vi "assign object ID.vi"(3 "object calculations (previous)":T2[](array[typedef]), 4 "robot location":cluster{"x":i16, "y":i16}, 5 "visible objects":T3[](array[typedef])) -> (0 "faulty trailer detection":bool, 2 "IDed objects":T1(array[cluster]))   [LabVIEW 2009]
uses:
  visible object.ctl
  object velocity and calculations.ctl
panel:
  out "checksum 2":i32
  out "checksum 1":i16
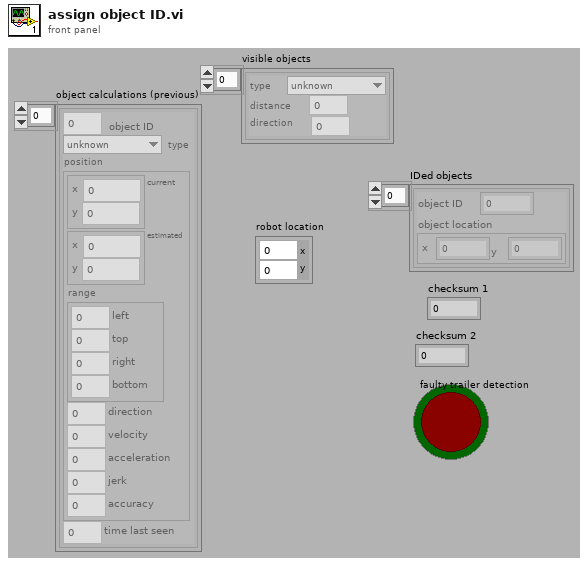
[diagram p1: front panel]
types:
  T1 = cluster{"object ID":i32, "object location":cluster{"x":dbl, "y":dbl}}[]
  T2 = typedef "object velocity and calculations.ctl" = cluster{"object ID":i32, "type":enum8{"unknown", "moonrock", "empty cell", "supercell", "target trailer"}, "position":cluster{"current":cluster{"x":dbl, "y":dbl}, "estimated":cluster{"x":dbl, "y":dbl}, "range":cluster{"left":dbl, "top":dbl, "right":dbl, "bottom":dbl}, "direction":dbl, "velocity":dbl, "acceleration":dbl, "jerk":dbl, "accuracy":dbl}, "time last seen":i32}
  T3 = typedef "visible object.ctl" = cluster{"type":enum8{"unknown", "moonrock", "empty cell", "supercell", "target trailer"}, "distance":dbl, "direction":dbl}
  T4 = enum8{"unknown", "moonrock", "empty cell", "supercell", "target trailer"}
  T5 = cluster{"current":cluster{"x":dbl, "y":dbl}, "estimated":cluster{"x":dbl, "y":dbl}, "range":cluster{"left":dbl, "top":dbl, "right":dbl, "bottom":dbl}, "direction":dbl, "velocity":dbl, "acceleration":dbl, "jerk":dbl, "accuracy":dbl}
  T6 = cluster{"left":dbl, "top":dbl, "right":dbl, "bottom":dbl}
  T7 = cluster{"In Range?":bool, "distance":dbl, i32, cluster{dbl, dbl}}
  T8 = cluster{"In Range?":bool, "distance":dbl, i32, cluster{dbl, dbl}}[]
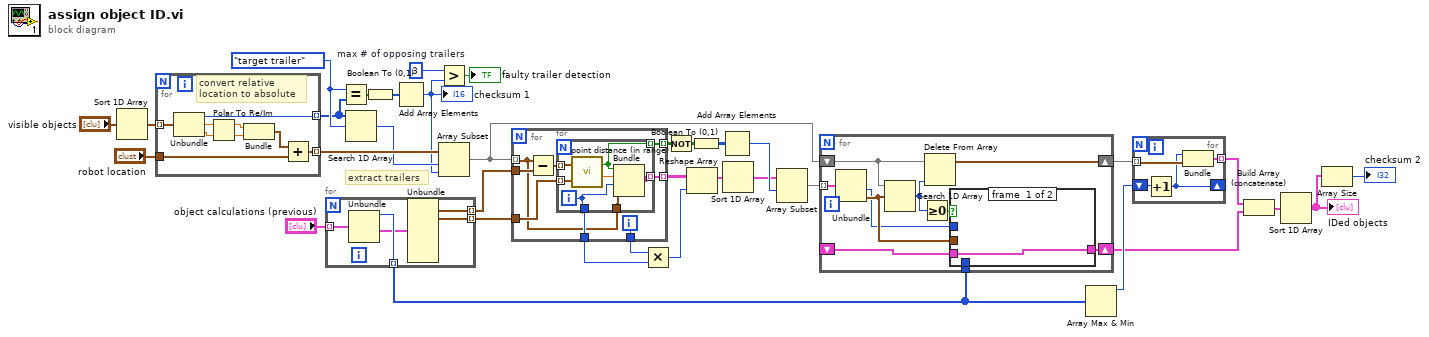
[diagram p0: block diagram]
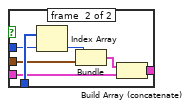
[diagram p2: hidden frame]
diagram:
  w26 = i16 3  # max # of opposing trailers
  w31 = T4."target trailer" ("type")
  # "extract trailers"
  n1 = Sort 1D Array(array="visible objects") -> (sorted array=w33:T3[])
  n2 = for {
    tunnel: w33 -> [w44] mode=indexing
    tunnel: "robot location" -> [w38]
    tunnel: [w37] -> w32 mode=indexing
    tunnel: [w36] -> w30 mode=indexing
    # "convert relative\nlocation to absolute"
    n3 = Unbundle(w44) -> ("type"=w36:T4, "distance"=w43:dbl, "direction"=w42:dbl)
    n4 = Polar To Re/Im(2:w42, 3:w43) -> (0:w41:dbl, 1:w40:dbl)
    n5 = Bundle(w40, w41) -> (w39:cluster{dbl, dbl})  [unwired: 1 in]
    n6 = Add(x=w39, y=w38) -> (x+y=w37:cluster{dbl, dbl})
  }
  n7 = for {
    tunnel: "object calculations (previous)" -> [w49] mode=indexing
    tunnel: [w48] -> w10 mode=indexing
    tunnel: [w46] -> w24 mode=indexing
    tunnel: [w45] -> w23 mode=indexing
    n8 = Unbundle(w49) -> ("object ID"=w48:i32, "position"=w47:T5)  [unwired: 2 out]
    n9 = Unbundle(w47) -> ("estimated"=w46:cluster{"x":dbl, "y":dbl}, "range"=w45:T6)  [unwired: 6 out]
  }
  n10 = Equal?(x=w31, y=w30) -> (x = y?=w29:bool[])
  n11 = Search 1D Array(1D array=w30, element=w31) -> (index of element=w27:i32)  [unwired: 1 in]
  n12 = Boolean To (0,1)(Boolean=w29) -> (0, 1=w28:i16[])
  n13 = Add Array Elements(numeric array=w28) -> (sum=w2:i16)
  "checksum 1" <- w2
  n14 = Greater?(x=w26, y=w2) -> (0:→"faulty trailer detection":bool)
  n15 = Array Subset(array=w32, index=w27, length=w2) -> (w11:cluster{dbl, dbl}[])
  n16 = for {
    tunnel: w11 -> [w50] mode=indexing
    tunnel: w24 -> [w57]
    tunnel: w23 -> [w55]
    tunnel: [w54] -> w20 mode=indexing
    tunnel: [w53] -> w21
    tunnel: [w51] -> w22
    tunnel: [w52] -> w16 mode=indexing
    i -> [w51]
    n17 = Subtract(x=w50, y=w57) -> (x-y=w56:cluster{dbl, dbl}[])
    n18 = for {
      tunnel: w56 -> [w63] mode=indexing
      tunnel: w55 -> [w64] mode=indexing
      tunnel: [w61] -> w54 mode=indexing
      tunnel: [w60] -> w52 mode=indexing
      tunnel: [w59] -> w53
      tunnel: w50 -> [w58]
      i -> [w59]
      n19 = call "point distance (in range).vi"("range"=w64, "cartesian location"=w63) -> ("distance"=w62:dbl, "In Range?"=w60:bool)
      n20 = Bundle("In Range?"=w60, "distance"=w62, w59, w58) -> (w61:T7)  [unwired: 1 in]
    }
  }
  n21 = Multiply(x=w22, y=w21) -> (x*y=w19:i32)
  n22 = Not(x=w16) -> (.not. x?=w18:bool[][])
  n23 = Reshape Array(w20, w19) -> (w15:T8)
  n24 = Boolean To (0,1)(Boolean=w18) -> (0, 1=w17:i16[][])
  n25 = Add Array Elements(numeric array=w17) -> (sum=w14:i16)
  n26 = Sort 1D Array(array=w15) -> (sorted array=w13:T8)
  n27 = Array Subset(array=w13, index=w14) -> (w12:T8)  [unwired: 1 in]
  n28 = for {
    tunnel: w12 -> [w74] mode=indexing
    shift-right: [w72] -> w8
    shift-left: w11 -> [w73]
    tunnel: w10 -> [w68]
    shift-right: [w66] -> w6
    shift-left: _ -> [w65]
    n29 = Unbundle(w74) -> (w67:i32, w69:cluster{dbl, dbl})  [unwired: 2 out]
    n30 = Search 1D Array(1D array=w73, element=w69) -> (index of element=w71:i32)  [unwired: 1 in]
    n31 = Greater Or Equal To 0?(x=w71) -> (x >= 0?=w70:bool)
    n32 = Delete From Array(array=w73, index=w71) -> (array with subset deleted=w72:cluster{dbl, dbl}[])  [unwired: 1 in, 1 out]
    n33 = case shown="True" w70 {
      tunnel: w69 -> [_ w79]
      tunnel: w68 -> [_ w82]
      tunnel: w67 -> [_ w81]
      tunnel: [w75 w77] -> w66
      tunnel: w65 -> [w75 w76]
      frame #0 {
      }
      frame #1 {
        n34 = Index Array(array=w82, index=w81) -> (element=w80:i32)
        n35 = Bundle("object ID"=w80, w79) -> (w78:cluster{"object ID":i32, cluster{dbl, dbl}})  [unwired: 1 in]
        n36 = Build Array (concatenate)(w78, w76) -> (w77:cluster{"object ID":i32, cluster{dbl, dbl}}[])
      }
    }
  }
  n37 = Array Max & Min(array=w10) -> (max value=w9:i32)  [unwired: 3 out]
  n38 = for {
    shift-right: [w84] -> _
    shift-left: w9 -> [w86]
    tunnel: w8 -> [w85] mode=indexing
    tunnel: [w83] -> w7 mode=indexing
    n39 = Increment(x=w86) -> (x+1=w84:i32)
    n40 = Bundle(w84, w85) -> (w83:cluster{i32, cluster{dbl, dbl}})  [unwired: 1 in]
  }
  n41 = Build Array (concatenate)(w7, w6) -> (w5:cluster{"object ID":i32, cluster{dbl, dbl}}[])
  n42 = Sort 1D Array(array=w5) -> (sorted array=w4:cluster{"object ID":i32, cluster{dbl, dbl}}[])
  "IDed objects" <- w4
  n43 = Array Size(array=w4) -> (size(s)=→"checksum 2":i32)
